vi "Display3DTrain.vi"(8 "error in":errorcluster, 11 "Local":T7={"Parameter"={"3D Plot"=[], "3D Scatter"=refnum, "Data"={"Split"={"X Train"=[], "X Test"=[], "Y Train"=[], "Y Test"=[]}, "Predict"=[]}, "Display"={"Choice"=enum."All", "Indexe"={"X"=0, "Y"=1, "Z"=2}}, "Point Property"={"Train Style"=enum."Full circle", "Test OK Style"=enum."Full square", "Label Color"=[8978528, 4367871, 1985280], "Test NO OK"={"Style"=enum."Cross", "Color"=16716800}}, "3D Plot Datatype.lvclass"=refnum}, "3DArray"=[], "Rating 3D Array"=[], "GoodPredict"=0, "Point ID"=[]}) -> (0 "error out":errorcluster, 3 "Local Out":T5)   [LabVIEW 2020]
doc: "Display 3D graph"
uses:
  _Controls/3DParameters.ctl
  <vilib>/Math Plots/3D Math Plots/3D Plot/3D Plot Datatype/3D Plot Datatype.lvclass
  <vilib>/Math Plots/3D Math Plots/3D Scatter/3D Scatter XCtrl/3D Scatter.xctl
  _Controls/Datas.ctl
  _Controls/PointPropertyMultipleLabel.ctl
  _Controls/Style.ctl
  _Controls/3DData.ctl
  <vilib>/Math Plots/3D Math Plots/3D Plot/3D Plot/Typedef/Color Ramp Cluster.ctl
  <vilib>/Math Plots/3D Math Plots/3D Plot/3D Plot/3D Plot.lvclass
types:
  T1 = typedef "Datas.ctl" = cluster{"Split":cluster{"X Train":dbl[][], "X Test":dbl[][], "Y Train":dbl[][], "Y Test":dbl[][]}, "Predict":dbl[][]}
  T2 = typedef "PointPropertyMultipleLabel.ctl" = cluster{"Train Style":T3, "Test OK Style":T3, "Label Color":u32[], "Test NO OK":cluster{"Style":T3, "Color":u32}}
  T3 = typedef "Style.ctl" = enum16{"Empty circle", "Full circle", "Empty square", "Full square", "Cross"}
  T4 = typedef "3DData.ctl" = cluster{"Tag":i32, "X":dbl[], "Y":dbl[], "Z":dbl[]}
  T5 = cluster{"Parameter":cluster{"3D Plot":refnum<class "3D Plot Datatype.lvclass">[], "3D Scatter":refnum<vi>, "Data":T1, "Display":cluster{"Choice":enum16{"All", "Train", "Test"}, "Indexe":cluster{"X":i32, "Y":i32, "Z":i32}}, "Point Property":T2, "3D Plot Datatype.lvclass":refnum<class "3D Plot Datatype.lvclass">}, "3DArray":cluster{"X":dbl[], "Y":dbl[], "Z":dbl[]}[], "Rating 3D Array":T4[], "GoodPredict":i32, "Point ID":cluster{"DataUse":enum16{"Dataset", "Train", "Test"}, "Color":u32}[]}
  T6 = typedef "3DParameters.ctl" = cluster{"3D Plot":refnum<class "3D Plot Datatype.lvclass">[], "3D Scatter":refnum<vi>, "Data":T1, "Display":cluster{"Choice":enum16{"All", "Train", "Test"}, "Indexe":cluster{"X":i32, "Y":i32, "Z":i32}}, "Point Property":T2, "3D Plot Datatype.lvclass":refnum<class "3D Plot Datatype.lvclass">}
  T7 = cluster{"Parameter":T6, "3DArray":cluster{"X":dbl[], "Y":dbl[], "Z":dbl[]}[], "Rating 3D Array":T4[], "GoodPredict":i32, "Point ID":cluster{"DataUse":enum16{"Dataset", "Train", "Test"}, "Color":u32}[]}
  T8 = typedef "3D Plot.lvclass/Color Ramp Cluster.ctl" = cluster{"Color Ramp Style":enum16{"None", "Shaded", "Color spectrum", "Grey scale", "Custom"}, "Color Ramp Array":u32[], "Color Ramp Index":i32[], "Interpolate?":bool, "Logarithm?":bool}
  T9 = cluster{"DataUse":enum16{"Dataset", "Train", "Test"}, "Color":u32}[]
  T10 = typedef "3D Plot.lvclass/Sprite Type.ctl" = enum16{"None", "Empty Square", "Solid Square", "Empty Diamond", "Solid Diamond", "Empty Circle", "Solid Circle", "Asterisk", "Bold X", "Wireframe Sphere", "Solid Sphere", "Wireframe Cube", "Solid Cube"}
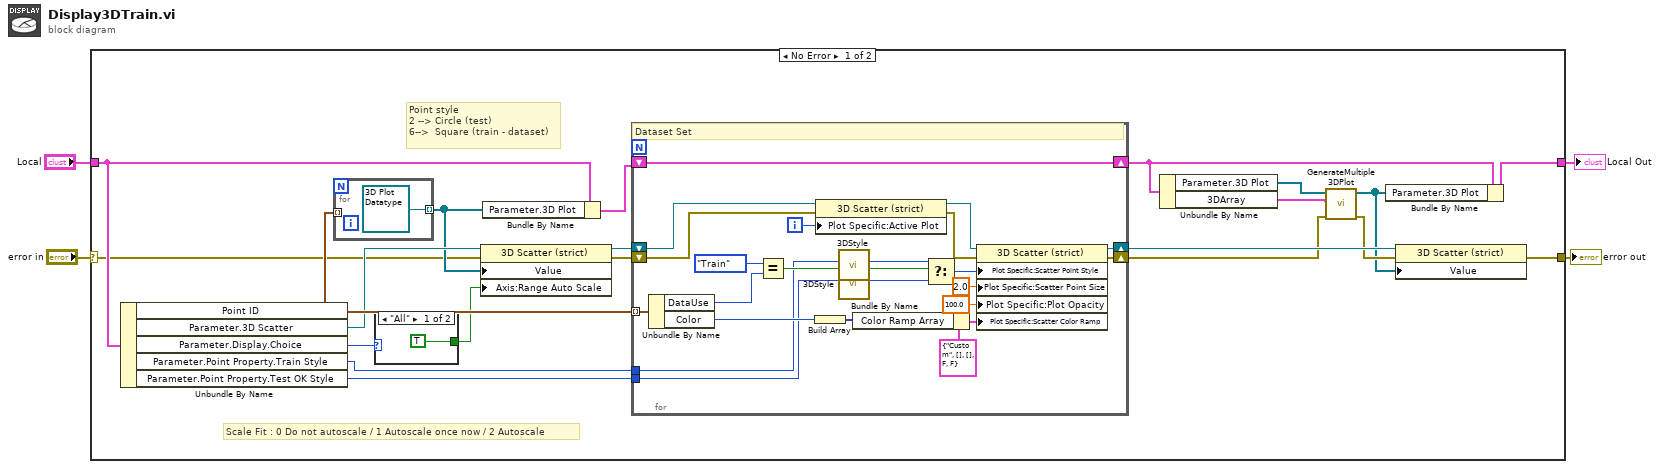
[diagram p0: block diagram]
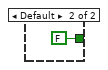
[diagram p2: hidden frame]
diagram:
  n1 = case shown="No Error" "error in" {
    selector: "error in" -> [w7 w53]
    tunnel: "Local" -> [w22 w52]
    tunnel: [w25 w53] -> w3
    tunnel: [w24 w52] -> w1
    frame No Error {
      # "Scale Fit : 0 Do not autoscale / 1 Autoscale once now / 2 Autoscale"
      # "Point style \n2 --> Circle (test)\n6-->  Square (train - dataset)"
      n2 = Unbundle By Name(w22) -> ("Point ID"=w23:T9, "Parameter.3D Scatter"=w10:refnum<vi>, "Parameter.Display.Choice"=w21:enum16{"All", "Train", "Test"}, "Parameter.Point Property.Train Style"=w6:T3, "Parameter.Point Property.Test OK Style"=w5:T3)
      n3 = for {
        tunnel: [refnum<class "3D Plot Datatype.lvclass"> refnum ("3D Plot Datatype.lvclass")] -> w9 mode=indexing
        tunnel: w23 -> [_] mode=indexing
      }
      n4 = case shown="\"All\"" w21 {
        tunnel: [TRUE ("x = y?") FALSE ("x = y?")] -> w8
        frame "All" {
        }
        frame Default {
        }
      }
      n5 = property class="3D Scatter (strict)"(reference=w10, error in=w7, "Value"=w9, "Axis:Range Auto Scale"=w8) -> (reference out=w20:refnum<vi>, error out=w17:errorcluster)
      n6 = Bundle By Name(cluster=w22, "Parameter.3D Plot"=w9) -> (w19:T7)
      n7 = for {
        tunnel: w23 -> [w48] mode=indexing
        shift-right: [w45] -> w18
        shift-left: w19 -> [w45]
        shift-right: [w43] -> w16
        shift-left: w20 -> [w42]
        shift-right: [w49] -> w13
        shift-left: w17 -> [w31]
        tunnel: w6 -> [w29]
        tunnel: w5 -> [w28]
        i -> [w40]
        # "Dataset Set"
        n8 = Unbundle By Name(w48) -> ("DataUse"=w46:enum16{"Dataset", "Train", "Test"}, "Color"=w38:u32)
        n9 = Equal?(x=enum16{"Dataset", "Train", "Test"}."Train", y=w46) -> (x = y?=w47:bool)
        n10 = Build Array(w38) -> (w37:u32[])
        n11 = property class="3D Scatter (strict)"(reference=w42, error in=w31, "Plot Specific:Active Plot"=w40) -> (reference out=w41:refnum<vi>, error out=w39:errorcluster)
        n12 = call "3DStyle.vi"("Style"=w29) -> ("Scatter Point Style"=w30:T10)  [unwired: 10 in]
        n13 = call "3DStyle.vi"("Style"=w28) -> ("Scatter Point Style"=w27:T10)  [unwired: 10 in]
        n14 = Bundle By Name(cluster=T8 {"Color Ramp Style"=enum."Custom", "Color Ramp Array"=[], "Color Ramp Index"=[], "Interpolate?"=FALSE, "Logarithm?"=FALSE} ("Spécifique à un tracé:Nuage:Rampe de couleur du nuage"), "Color Ramp Array"=w37) -> (w35:T8)
        n15 = Select(t=w30, s=w47, f=w27) -> (s? t:f=w32:T10)
        n16 = property class="3D Scatter (strict)"(reference=w41, error in=w39, "Plot Specific:Scatter Point Style"=w32, "Plot Specific:Scatter Point Size"=sgl 2.0 ("Plot Specific:Scatter:Scatter Point Size"), "Plot Specific:Plot Opacity"=sgl 100.0 ("Plot Specific:General:Plot Opacity"), "Plot Specific:Scatter Color Ramp"=w35) -> (reference out=w43:refnum<vi>, error out=w49:errorcluster)
      }
      n17 = Unbundle By Name(w18) -> ("Parameter.3D Plot"=w15:refnum<class "3D Plot Datatype.lvclass">[], "3DArray"=w14:cluster{"X":dbl[], "Y":dbl[], "Z":dbl[]}[])
      n18 = call "GenerateMultiple3DPlot.vi"("error in"=w13, "3D Array"=w14, "3D Scatter"=w15) -> ("error out"=w12:errorcluster, "3D Scatter Out"=w11:refnum<class "3D Plot Datatype.lvclass">[])  [unwired: 7 in]
      n19 = Bundle By Name(cluster=w18, "Parameter.3D Plot"=w11) -> (w24:T7)
      n20 = property class="3D Scatter (strict)"(reference=w16, error in=w12, "Value"=w11) -> (error out=w25:errorcluster)  [unwired: 1 out]
    }
    frame Error {
    }
  }
  "error out" <- w3
  "Local Out" <- w1
